vi "Read Recurrence Interval (s).vi"(8 "error in (no error)":errorcluster, 11 "AExpense in":refnum<class "AExpense.lvclass">) -> (0 "error out":errorcluster, 2 "Recurrence Interval (s)":u32, 3 "AExpense out":refnum<class "AExpense.lvclass">)   [LabVIEW 2020, in "AExpense.lvclass"]
uses:
  AExpense.lvclass
  AExpense.lvclass/AExpense.ctl
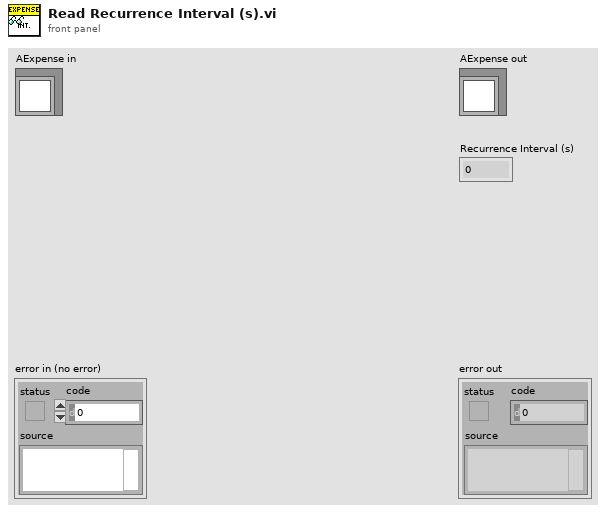
[diagram p1: front panel]
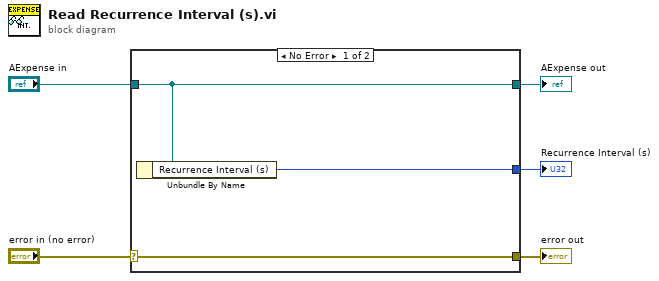
[diagram p0: block diagram]
diagram:
  n1 = case shown="No Error" "error in (no error)" {
    selector: "error in (no error)" -> [w8 w9]
    tunnel: [w8 w9] -> w4
    tunnel: [w7 w10] -> w2
    tunnel: "AExpense in" -> [w7 w10]
    tunnel: [w6 _] -> w1
    frame No Error {
      n2 = Unbundle By Name(w7) -> ("Recurrence Interval (s)"=w6:u32)
    }
    frame Error {
    }
  }
  "error out" <- w4
  "AExpense out" <- w2
  "Recurrence Interval (s)" <- w1
